vi "setAuthority.vi"(8 "error in (no error)":errorcluster, 10 "Num of Bending Mode":i32=20, 11 "OptCtrl in":refnum<class "OptCtrl.lvclass">) -> (0 "error out":errorcluster, 3 "OptCtrl out":refnum<class "OptCtrl.lvclass">)   [LabVIEW 2016, in "OptCtrl.lvclass"]
doc: "Set the authority of subsystems. The penality is considered. The array order is [M2 hexapod, camera hexapod, M1M3 bending mode, M2 bending mode]."
uses:
  OptCtrl.lvclass
  OptCtrl.lvclass/OptCtrl.ctl
panel:
  in  "M2 Subsystem":T1={"Mirror"="M2", "Actuatro Force File"="M2_1um_force.DAT"}
  in  "M1M3 Subsystem":T1={"Mirror"="M1M3", "Actuatro Force File"="M1M3_1um_156_force.DAT"}
  in  "Rigid Body Stroke File":string="rbStroke.txt"
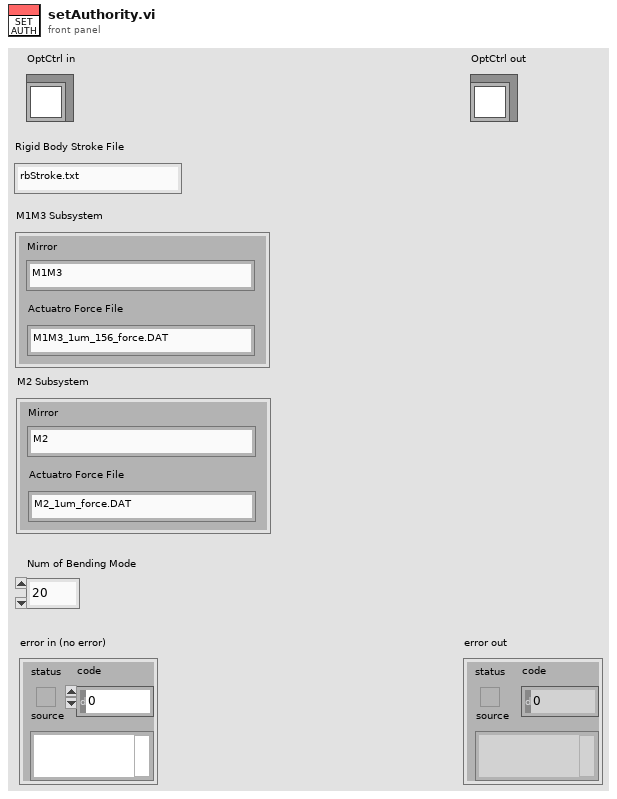
[diagram p1: front panel]
types:
  T1 = cluster{"Mirror":string, "Actuatro Force File":string}
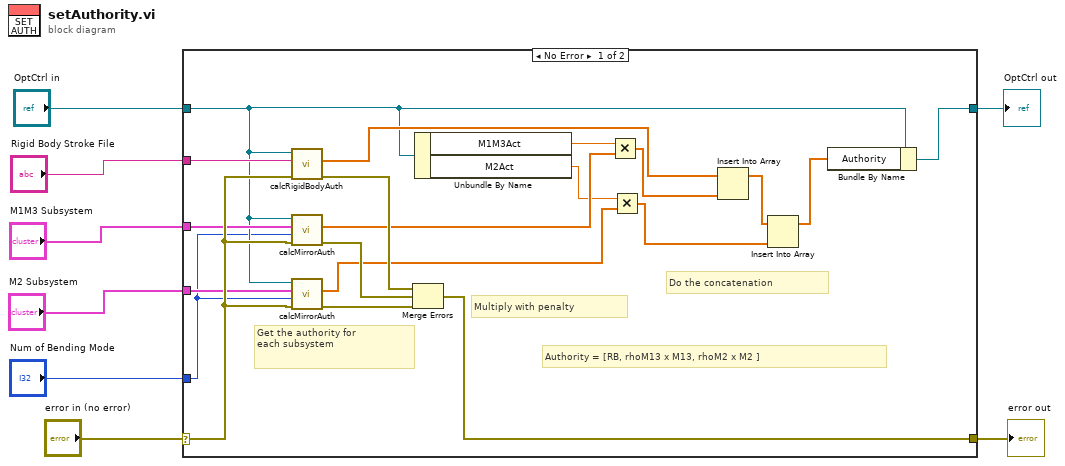
[diagram p0: block diagram]
diagram:
  n1 = case shown="No Error" "error in (no error)" {
    selector: "error in (no error)" -> [w28 w30]
    tunnel: [w24 w30] -> w7
    tunnel: [w10 w29] -> w6
    tunnel: "OptCtrl in" -> [w11 w29]
    tunnel: "Rigid Body Stroke File" -> [w23 _]
    tunnel: "M1M3 Subsystem" -> [w22 _]
    tunnel: "M2 Subsystem" -> [w21 _]
    tunnel: "Num of Bending Mode" -> [w9 _]
    frame No Error {
      # "Authority = [RB, rhoM13 x M13, rhoM2 x M2 ]"
      # "Do the concatenation"
      # "Multiply with penalty"
      # "Get the authority for \neach subsystem"
      n2 = call "calcRigidBodyAuth.vi"("error in (no error)"=w28, "Rigid Body Stroke File"=w23, "OptCtrl in"=w11) -> ("error out"=w27:errorcluster, "Authority (1 um)"=w16:dbl[])  [unwired: 6 in, 1 out]
      n3 = call "calcMirrorAuth.vi"("error in (no error)"=w28, "Num of Bending Mode"=w9, "Subsystem"=w22, "OptCtrl in"=w11) -> ("error out"=w26:errorcluster, "Authority (1 N RMS)"=w19:dbl[])  [unwired: 5 in, 1 out]
      n4 = call "calcMirrorAuth.vi"("error in (no error)"=w28, "Num of Bending Mode"=w9, "Subsystem"=w21, "OptCtrl in"=w11) -> ("error out"=w25:errorcluster, "Authority (1 N RMS)"=w17:dbl[])  [unwired: 5 in, 1 out]
      n5 = Merge Errors(w27, w26, w25) -> (w24:errorcluster)
      n6 = Unbundle By Name(w11) -> ("M1M3Act"=w20:dbl, "M2Act"=w18:dbl)
      n7 = Multiply(x=w20, y=w19) -> (x*y=w15:dbl[])
      n8 = Multiply(x=w18, y=w17) -> (x*y=w13:dbl[])
      n9 = Insert Into Array(array=w16, new element=w15) -> (w14:dbl[])  [unwired: 1 in]
      n10 = Insert Into Array(array=w14, new element=w13) -> (w12:dbl[])  [unwired: 1 in]
      n11 = Bundle By Name(cluster=w11, "Authority"=w12) -> (w10:refnum<class "OptCtrl.lvclass">)
    }
    frame Error {
    }
  }
  "error out" <- w7
  "OptCtrl out" <- w6
